vi "Not Touched.vi"(11 "number":i32) -> (3 "not touched":bool)   [LabVIEW 2017, in "NI_Robotics_AnytimeDStar.lvclass"]
uses:
  <vilib>/robotics/Navigation/Anytime D Star/NI_Robotics_AnytimeDStar.lvclass
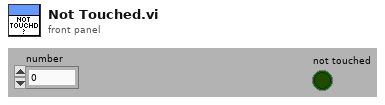
[diagram p1: front panel]
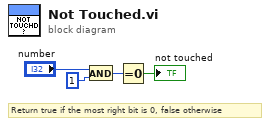
[diagram p0: block diagram]
diagram:
  # "Return true if the most right bit is 0, false otherwise"
  n1 = And(x="number", y=1) -> (x .and. y?=w2:i32)
  n2 = Equal To 0?(x=w2) -> (x = 0?=→"not touched":bool)
